vi "Build2dMap.vi"(0 "2D in":picture, 1 "new listing":string[][](table), 2 "Mod":T1=enum."Bounce", 3 "Desired Dimensions":cluster{"Width":i32, "Height":i32}, 4 "Old listing":string[][](table)) -> (5 "2D Map":picture, 6 "changed?":bool, 7 "LUT":T2(array[cluster]))   [LabVIEW 2012]
uses:
  SlideParams.ctl
  LVPresent_Globals.vi
panel:
  out "first time?":bool
  out "Array":bool[][](array[boolean])
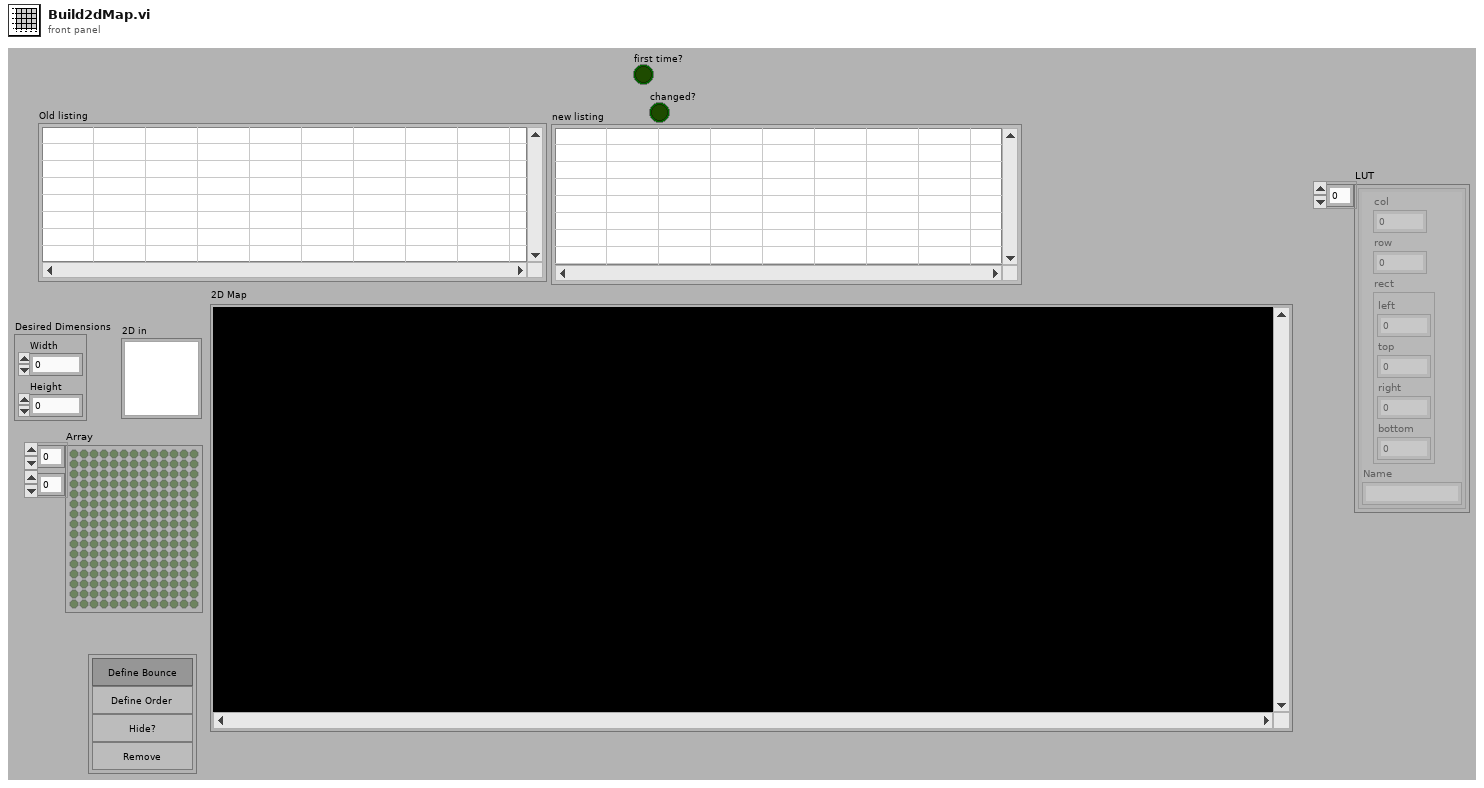
[diagram p1: front panel]
types:
  T1 = typedef "SlideParams.ctl" = enum32{"No Selection", "Bounce", "Order", "Hide", "Remove"}
  T2 = cluster{"col":i32, "row":i32, "rect":cluster{"left":i16, "top":i16, "right":i16, "bottom":i16}, "Name":string}[]
  T3 = cluster{"left":i16, "top":i16, "right":i16, "bottom":i16}
  T4 = cluster{i32, i32, "frame":cluster{"left":i16, "top":i16, "right":i16, "bottom":i16}, string}
  T5 = cluster{"col":i32, "row":i32, "frame":cluster{"left":i16, "top":i16, "right":i16, "bottom":i16}, "Name":string}[]
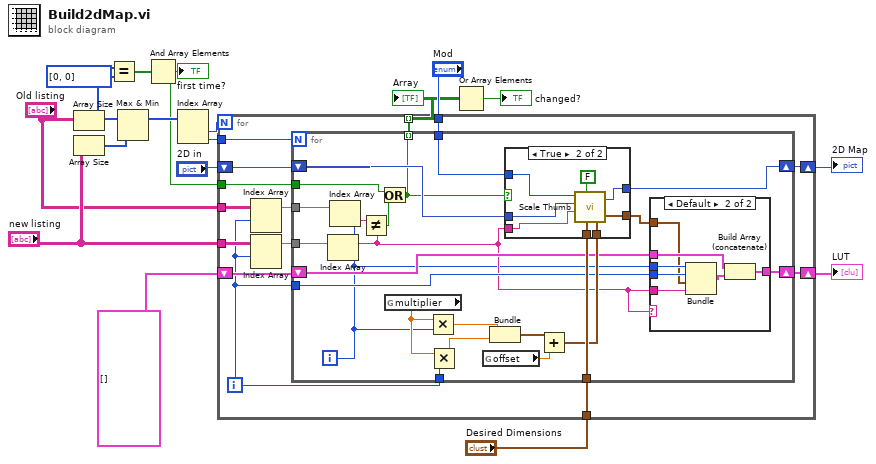
[diagram p0: block diagram]
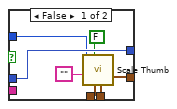
[diagram p3: hidden frame]
diagram:
  n1 = Array Size(array="Old listing") -> (size(s)=w2:i32[])
  n2 = Array Size(array="new listing") -> (size(s)=w12:i32[])
  n3 = Equal?(x=w2, y=i32[] [0, 0]) -> (x = y?=w4:bool[])
  n4 = Max & Min(x=w2, y=w12) -> (max(x,y)=w11:i32[])  [unwired: 1 out]
  n5 = And Array Elements(Boolean array=w4) -> (logical AND=w3:bool)
  "first time?" <- w3
  n6 = Index Array(array=w11) -> (element #1=w10:i32, element #2=w9:i32)  [unwired: 2 in]
  n7 = for {
    N: w10 -> [_]
    tunnel: "new listing" -> [w32]
    shift-right: [w30] -> w13
    shift-left: "2D in" -> [w31]
    tunnel: "Desired Dimensions" -> [w29]
    shift-right: [w28] -> w16
    shift-left: T2 [] ("LUT") -> [w27]
    tunnel: "Mod" -> [w26]
    tunnel: "Old listing" -> [w25]
    tunnel: [w24] -> w7 mode=indexing
    tunnel: w9 -> [w23]
    tunnel: w3 -> [w19]
    i -> [w20]
    n8 = Index Array(array=w25, index (row)=w20) -> (element=w22:string[])  [unwired: 1 in]
    n9 = Index Array(array=w32, index (row)=w20) -> (element=w21:string[])  [unwired: 1 in]
    n10 = for {
      N: w23 -> [_]
      tunnel: w21 -> [w42]
      shift-right: [w51] -> w30
      shift-left: w31 -> [w55]
      tunnel: w20 -> [w54]
      tunnel: w29 -> [w50]
      tunnel: w20 -> [w47]
      shift-right: [w45] -> w28
      shift-left: w27 -> [w46]
      tunnel: w26 -> [w44]
      tunnel: w22 -> [w39]
      tunnel: [w33] -> w24 mode=indexing
      tunnel: w19 -> [w34]
      i -> [w36]
      n11 = Index Array(array=w42, index=w36) -> (element=w37:string)
      n12 = Index Array(array=w39, index=w36) -> (element=w38:string)
      n13 = Not Equal?(x=w38, y=w37) -> (x != y?=w35:bool)
      n14 = Or(x=w34, y=w35) -> (x .or. y?=w33:bool)
      n15 = global read "LVPresent_Globals.vi" "multiplier"() -> (w40:sgl)
      n16 = Multiply(x=w40, y=w36) -> (x*y=w52:sgl)
      n17 = Multiply(x=w40, y=w54) -> (x*y=w53:sgl)
      n18 = global read "LVPresent_Globals.vi" "offset"() -> (w41:sgl)
      n19 = Bundle(w52, w53) -> (w49:cluster{sgl, sgl})  [unwired: 1 in]
      n20 = Add(x=w49, y=w41) -> (x+y=w48:cluster{sgl, sgl})
      n21 = case shown="True" w33 {
        tunnel: w55 -> [w70 w78]
        tunnel: [w70 w77] -> w51
        tunnel: w50 -> [w68 w76]
        tunnel: w48 -> [w69 w75]
        tunnel: w44 -> [w65 w74]
        tunnel: w37 -> [_ w72]
        tunnel: [w67 w73] -> w43
        frame False {
          n22 = call "Scale Thumb.vi"("Desired Dimensions"=w68, "Full Size"=FALSE, "Offset"=w69, "file"="", "Mod"=w65) -> ("frame"=w67:T3)  [unwired: 1 in, 1 out]
        }
        frame True {
          n23 = call "Scale Thumb.vi"("Desired Dimensions"=w76, "Full Size"=FALSE, "Offset"=w75, "file"=w72, "picture in"=w78, "Mod"=w74) -> ("frame"=w73:T3, "new picture"=w77:picture)
        }
      }
      n24 = case shown="Default" w37 {
        tunnel: w36 -> [_ w63]
        tunnel: w47 -> [_ w62]
        tunnel: w46 -> [w56 w61]
        tunnel: [w56 w60] -> w45
        tunnel: w37 -> [_ w59]
        tunnel: w43 -> [_ w58]
        frame "" {
        }
        frame Default {
          n25 = Bundle(w63, w62, "frame"=w58, w59) -> (w57:T4)  [unwired: 1 in]
          n26 = Build Array (concatenate)(w61, w57) -> (w60:T5)
        }
      }
    }
  }
  "LUT" <- w16
  "Array" <- w7
  "2D Map" <- w13
  n27 = Or Array Elements(Boolean array=w7) -> (logical OR=→"changed?":bool)
